vi "Preview.vi"(8 "error in (no error)":errorcluster, 11 "input cluster":T1) -> (0 "error out":errorcluster)   [LabVIEW 2013, in "Simple Sequence Editor.lvlib"]
uses:
  Simple Sequence Editor.lvlib
  Types/StateVariables.ctl
  Types/ChannelProperties.ctl
  <vilib>/Analysis/1siggen.llb/Ramp Pattern by Samples.vi
  <vilib>/Analysis/1siggen.llb/Ramp Pattern by Delta.vi
  <vilib>/Analysis/NI_AALBase.lvlib
panel:
  out "System Waveform Graph":waveform(dbl)[](graph)
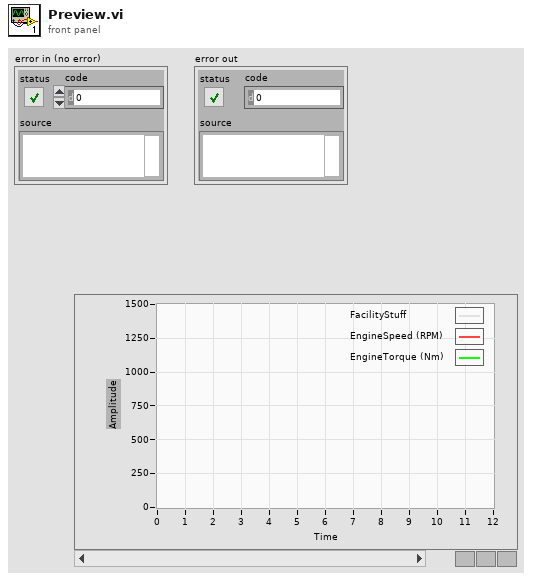
[diagram p1: front panel]
types:
  T1 = typedef "Simple Sequence Editor.lvlib/StateVariables.ctl" = cluster{"Aliases.All":T2[], "Aliases.Outputs":T2[], "UI.Sequence#ofColumns":i32, "SysDef.Path":path, "UI.SequenceRef":refnum<vi>}
  T2 = typedef "Simple Sequence Editor.lvlib/ChannelProperties.ctl" = cluster{"Name":string, "NodePath":string, "ScaleUnits":string}
  T3 = typedef "Simple Sequence Editor.lvlib/StepTypes.ctl" = enum8{"Step", "iStep", "Ramp", "Unchanged", "Unknown"}
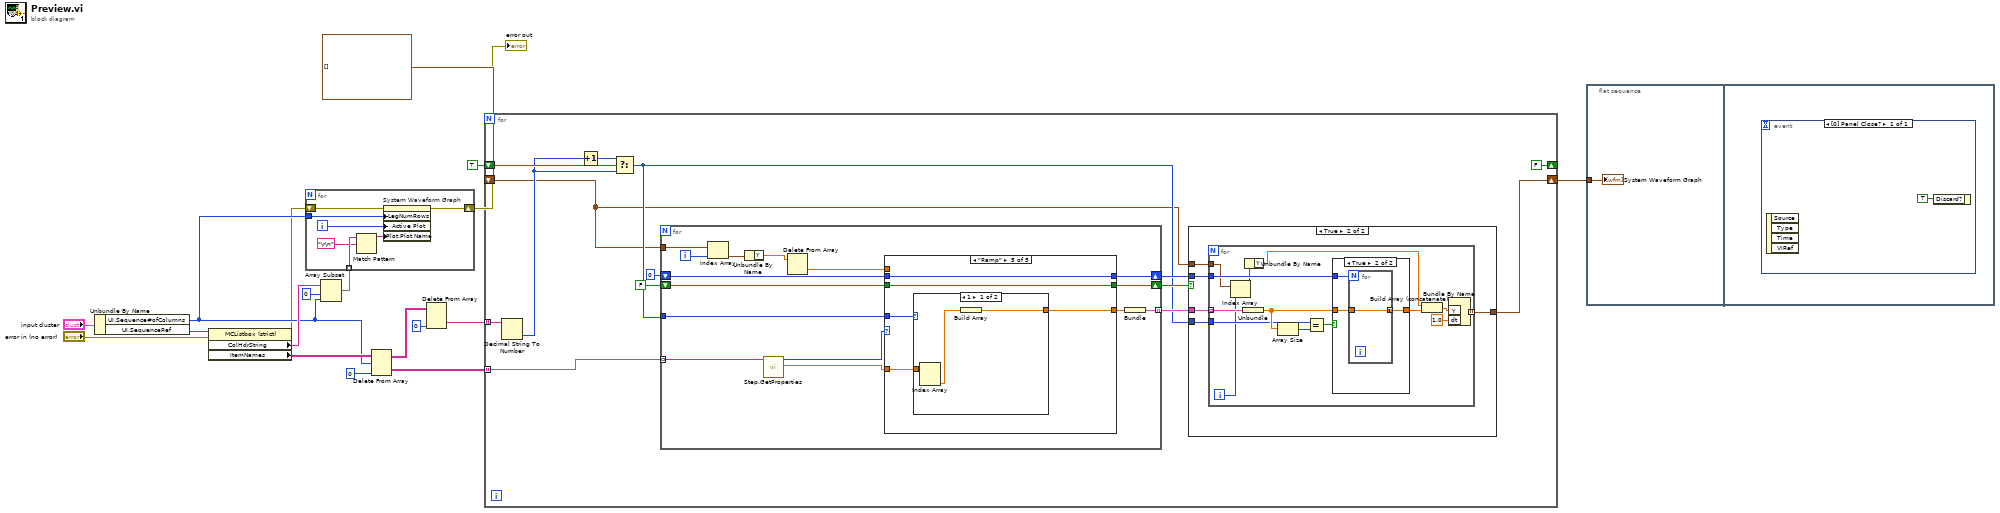
[diagram p0: block diagram]
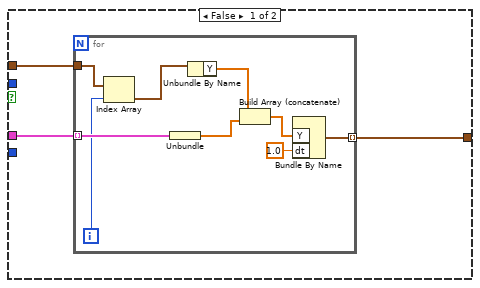
[diagram p2: hidden frame]
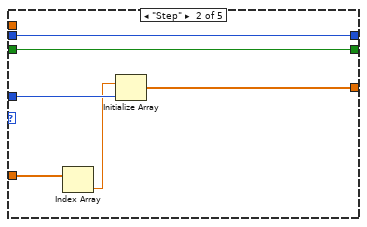
[diagram p5: hidden frame]
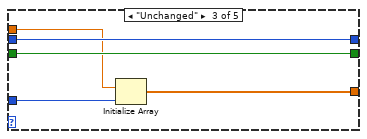
[diagram p6: hidden frame]
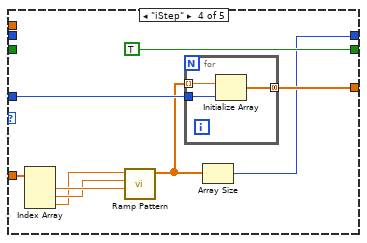
[diagram p7: hidden frame]
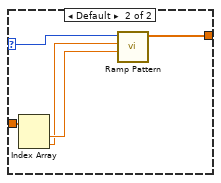
[diagram p8: hidden frame]
diagram:
  n1 = Unbundle By Name("input cluster") -> ("UI.Sequence#ofColumns"=w5:i32, "UI.SequenceRef"=w18:refnum<vi>)
  n2 = property class="MCListbox (strict)"(reference=w18, error in="error in (no error)") -> (error out=w2:errorcluster, "ColHdrString"=w6:string[], "ItemNames"=w7:string[][])  [unwired: 1 out]
  n3 = Array Subset(array=w6, index=0, length=w5) -> (w3:string[])
  n4 = for {
    tunnel: w5 -> [w25]
    tunnel: w3 -> [w22] mode=indexing
    shift-right: [w19] -> w1
    shift-left: w2 -> [w20]
    i -> [w24]
    n5 = Match Pattern(string=w22, regular expression="\r\n") -> (before substring=w23:string)  [unwired: 1 in, 3 out]
    n6 = property on="System Waveform Graph" class="WFGraph (strict)"(error in=w20, "LegNumRows"=w25, "Active Plot"=w24, "Plot.Plot Name"=w23) -> (error out=w19:errorcluster)  [unwired: 1 in, 1 out]
  }
  "error out" <- w1
  n7 = Delete From Array(array=w7, length=w5, index (col)=0 ("disabled index (col)")) -> (deleted portion=w15:string[][], array with subset deleted=w14:string[][])  [unwired: 1 in]
  n8 = Delete From Array(array=w14, index (col)=0 ("disabled index (col)")) -> (deleted portion=w13:string[])  [unwired: 2 in, 1 out]
  n9 = for {
    tunnel: w15 -> [w39] mode=indexing
    tunnel: w13 -> [w38] mode=indexing
    shift-right: [FALSE] -> _
    shift-left: TRUE -> [w31]
    shift-right: [w27] -> w9
    shift-left: waveform(dbl)[] [] -> [w26]
    n10 = Decimal String To Number(string=w38) -> (number=w30:i32)  [unwired: 2 in, 1 out]
    n11 = Increment(x=w30) -> (x+1=w29:i32)
    n12 = Select(t=w29, s=w31, f=w30) -> (s? t:f=w28:i32)
    n13 = for {
      tunnel: w39 -> [w90] mode=indexing
      tunnel: w28 -> [w88]
      shift-right: [w85] -> w35
      shift-left: FALSE -> [w86]
      shift-right: [w83] -> w34
      shift-left: 0 -> [w82]
      tunnel: [w81] -> w33 mode=indexing
      tunnel: w26 -> [w80]
      i -> [w78]
      n14 = Index Array(array=w80, index=w78) -> (element=w77:waveform(dbl))
      n15 = Unbundle By Name(w77) -> ("Y"=w76:dbl[])
      n16 = call "Step.GetProperties.vi"("String in"=w90) -> ("Parameters"=w87:dbl[], "Step"=w89:T3)  [unwired: 9 in]
      n17 = Delete From Array(array=w76) -> (deleted portion=w79:dbl)  [unwired: 2 in, 1 out]
      n18 = case shown="\"Ramp\"" w89 {
        tunnel: w88 -> [_ w98 w103 w111 w116]
        tunnel: w87 -> [_ w97 _ w112 w120]
        tunnel: [_ w95 w102 w106 w119] -> w84
        tunnel: w86 -> [w92 w94 w101 _ w118]
        tunnel: [w92 w94 w101 TRUE w118] -> w85
        tunnel: [w91 w93 w100 w104 w117] -> w83
        tunnel: w82 -> [w91 w93 w100 _ w117]
        tunnel: w79 -> [_ _ w99 _ _]
        frame Default {
        }
        frame "Step" {
          n19 = Index Array(array=w97) -> (element=w96:dbl)  [unwired: 1 in]
          n20 = Initialize Array(w96, w98) -> (w95:dbl[])
        }
        frame "Unchanged" {
          n21 = Initialize Array(w99, w103) -> (w102:dbl[])
        }
        frame "iStep" {
          n22 = Index Array(array=w112) -> (element #1=w110:dbl, element #2=w109:dbl, element #3=w108:dbl)  [unwired: 3 in]
          n23 = call-poly <vilib>:"Ramp Pattern.vi"("start"=w110, "end"=w109, "delta"=w108) -> ("Ramp Pattern"=w105:dbl[])  [unwired: 6 in, 2 out]
          n24 = for {
            tunnel: w111 -> [w115]
            tunnel: w105 -> [w114] mode=indexing
            tunnel: [w113] -> w106 mode=concatenating
            n25 = Initialize Array(w114, w115) -> (w113:dbl[])
          }
          n26 = Array Size(array=w105) -> (size(s)=w104:i32)
        }
        frame "Ramp" {
          n27 = case shown="1" w116 {
            selector: w116 -> [_ w124]
            tunnel: w120 -> [w123 w128]
            tunnel: [w121 w125] -> w119
            frame 1 {
              n28 = Index Array(array=w123) -> (element #2=w122:dbl)  [unwired: 2 in, 1 out]
              n29 = Build Array(w122) -> (w121:dbl[])
            }
            frame Default {
              n30 = Index Array(array=w128) -> (element #1=w127:dbl, element #2=w126:dbl)  [unwired: 2 in]
              n31 = call-poly <vilib>:"Ramp Pattern.vi"("start"=w127, "end"=w126, "samples"=w124) -> ("Ramp Pattern"=w125:dbl[])  [unwired: 7 in, 1 out]
            }
          }
        }
      }
      n32 = Bundle("Ramp Pattern"=w84) -> (w81:cluster{"Ramp Pattern":dbl[]})  [unwired: 1 in]
    }
    n33 = case shown="True" w35 {
      tunnel: w34 -> [_ w55]
      tunnel: w33 -> [w42 w56]
      tunnel: w28 -> [_ w54]
      tunnel: [w41 w53] -> w27
      tunnel: w26 -> [w40 w52]
      frame False {
        n34 = for {
          tunnel: w42 -> [w51] mode=indexing
          tunnel: [w49] -> w41 mode=indexing
          tunnel: w40 -> [w44]
          i -> [w45]
          n35 = Index Array(array=w44, index=w45) -> (element=w43:waveform(dbl))
          n36 = Unbundle(w51) -> ("Ramp Pattern"=w48:dbl[])
          n37 = Unbundle By Name(w43) -> ("Y"=w46:dbl[])
          n38 = Build Array (concatenate)(w46, w48) -> (w47:dbl[])
          n39 = Bundle By Name("Y"=w47, "dt"=1.0) -> (w49:waveform(dbl))  [unwired: 1 in]
        }
      }
      frame True {
        n40 = for {
          tunnel: w56 -> [w69] mode=indexing
          tunnel: w55 -> [w70]
          tunnel: w54 -> [w66]
          tunnel: [w63] -> w53 mode=indexing
          tunnel: w52 -> [w58]
          i -> [w59]
          n41 = Index Array(array=w58, index=w59) -> (element=w57:waveform(dbl))
          n42 = Unbundle(w69) -> ("Ramp Pattern"=w68:dbl[])
          n43 = Unbundle By Name(w57) -> ("Y"=w60:dbl[])
          n44 = Array Size(array=w68) -> (size(s)=w67:i32)
          n45 = Equal?(x=w66, y=w67) -> (x = y?=w65:bool)
          n46 = case shown="True" w65 {
            tunnel: w70 -> [_ w74]
            tunnel: w68 -> [w71 w73]
            tunnel: [w71 w72] -> w62
            frame False {
            }
            frame True {
              n47 = for {
                N: w74 -> [_]
                tunnel: w73 -> [w75]
                tunnel: [w75] -> w72 mode=concatenating
              }
            }
          }
          n48 = Build Array (concatenate)(w60, w62) -> (w61:dbl[])
          n49 = Bundle By Name("Y"=w61, "dt"=1.0) -> (w63:waveform(dbl))  [unwired: 1 in]
        }
      }
    }
  }
  n50 = flat-sequence {
    tunnel: w9 -> [w129]
    frame #0 {
      "System Waveform Graph" <- w129
    }
    frame #1 {
      n51 = event shown="[0] Panel Close?" {
        selector: _ -> [_]
        dyn-events: _ -> [_]
        timeout: _ -> [_]
        event Panel Close? {
          n52 = event-data() -> ()  [unwired: 1 in, 4 out]
          n53 = event-data("Discard?"=TRUE) -> ()  [unwired: 1 in, 1 out]
        }
      }
    }
  }
